vi "DSF.Engine.Plugin.Rx.Transfer Group.Move Data.vi"(8 "error in (no error)":errorcluster, 10 "Transfer Group in":refnum<class "DSF.Engine.Transfer Group.lvclass">, 11 "Plugin in":refnum<class "DSF.Engine.Plugin.lvclass">) -> (0 "error out":errorcluster, 2 "Transfer Group out":refnum<class "DSF.Engine.Transfer Group.lvclass">, 3 "Plugin out":refnum<class "DSF.Engine.Plugin.lvclass">)   [LabVIEW 2017, in "DSF.Engine.lvlib" / "DSF.Engine.Plugin.lvclass"]
uses:
  DSF.Engine.Plugin.lvclass
  Transfer/DSF.Engine.Transfer Group.lvclass
  Transfer/DSF.Engine.Transfer Group.lvclass/DSF.Engine.Transfer Group.ctl
  Transfer/DSF.Engine.Transfer.lvclass/DSF.Engine.Transfer.ctl
  Transfer/DSF.Engine.Transfer Group.Get Transfers.vi
  Transfer/DSF.Engine.Transfer.Get Inline Buffer.vi
  Transfer/DSF.Engine.Transfer.Get Intermediate Buffer.vi
  Built/Memory/Memory Manager.lvlibp/1abvi3w/vi.lib/National Instruments/Memory Manager/Classes/Pointer/Memory.Pointer.Copy All.vi
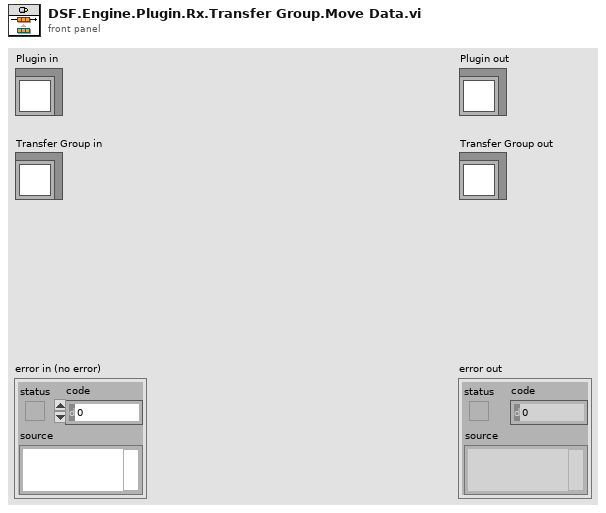
[diagram p1: front panel]
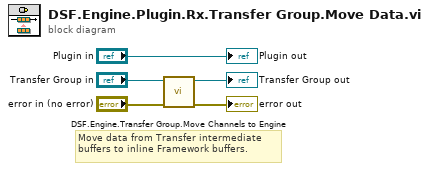
[diagram p0: block diagram]
diagram:
  # "Move data from Transfer intermediate buffers to inline Framework buffers."
  n1 = call "DSF.Engine.Transfer Group.Move Channels to Engine.vi"("error in (no error)"="error in (no error)", "Transfer Group in"="Transfer Group in") -> ("error out"=→"error out":errorcluster, "Transfer Group out"=→"Transfer Group out":refnum<class "DSF.Engine.Transfer Group.lvclass">)  [unwired: 8 in]
  "Plugin out" <- "Plugin in"
